vi "XGT 연속읽기 (독립).vi"() -> ()   [LabVIEW 2014]
uses:
  <vilib>/Instr/_visa.llb/VISA Configure Serial Port (Instr).vi
panel:
  out "error out":errorcluster
  in  "Start":bool
  out "배열":i32[](array[numeric])
  out "Array":i32[](array[numeric])
  in  "Address":string[](array[string])
  in  "length":i32=6
  out "데이터 개수":string
  out "에러 코드":string
  out "Waveform Graph":dbl[](graph)
  out "Serial Settings:Number of Bytes at Serial Port":u32
  in  "stop bits (10: 1 bit)":u16(ring)=10 caption="정지 비트(10: 1비트)" items=["1.0"=10, "1.5"=15, "2.0"=20]
  in  "parity (0:none)":enum16{"None", "Odd", "Even", "Mark", "Space"}(ring) caption="패리티(0:없음)"
  in  "data bits (8)":u16=8 caption="데이터 비트(8)" min=5 max=8 step=1
  in  "baud rate (9600)":u32=115200 caption="보 전송속도(9600)"
  in  "VISA resource name":refnum<visa-resource-name>="COM4" caption="VISA 리소스 이름"
  # "응답"
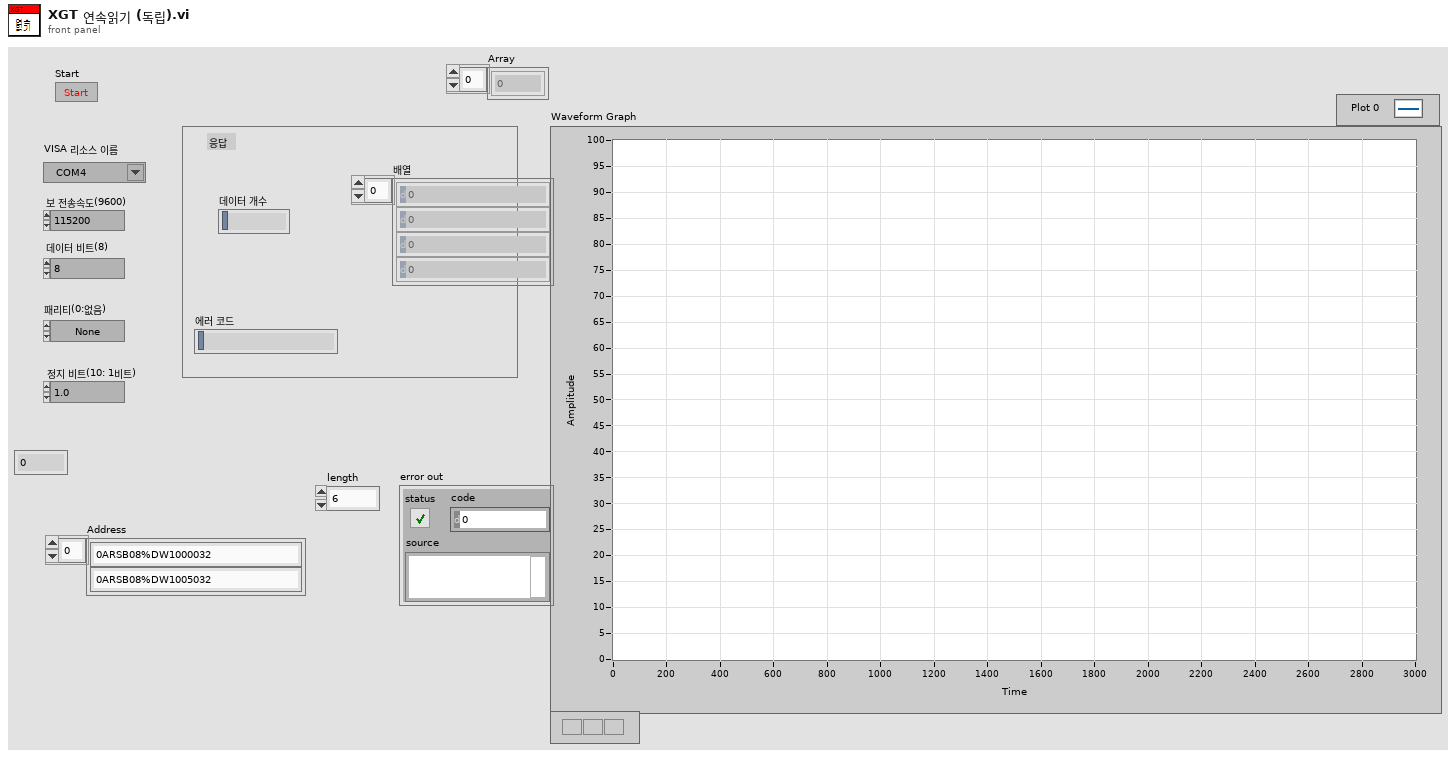
[diagram p1: front panel]
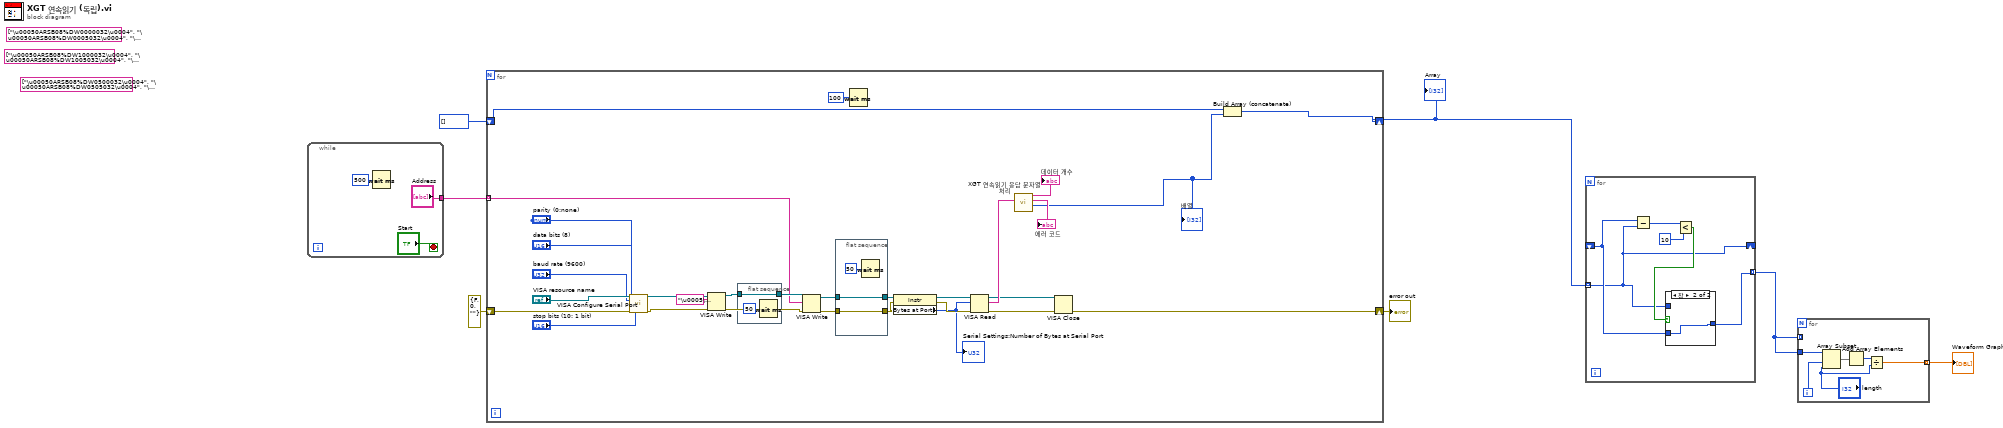
[diagram p0: block diagram]
diagram:
  (unwired) string[] ["\u00050ARSB08%DW1000032\u0004", "\u00050ARSB08%DW1005032\u0004", "\u00050ARSB08%DW1010032\u0004", "\u00050ARSB08%DW1015032\u0004", "\u00050ARSB08%DW1020032\u0004", "\u00050ARSB08%DW1025032\u0004", "\u00050ARSB08%DW1030032\u0004", "\u00050ARSB08%DW1035032\u0004", "\u00050ARSB08%DW1040032\u0004", "\u00050ARSB08%DW1045032\u0004", "\u00050ARSB08%DW1050032\u0004", "\u00050ARSB08%DW1055032\u0004", "\u00050ARSB08%DW1060032\u0004", "\u00050ARSB08%DW1065032\u0004", "\u00050ARSB08%DW1070032\u0004", "\u00050ARSB08%DW1075032\u0004", "\u00050ARSB08%DW1080032\u0004", "\u00050ARSB08%DW1085032\u0004", "\u00050ARSB08%DW1090032\u0004", "\u00050ARSB08%DW1095032\u0004", "\u00050ARSB08%DW1100032\u0004", "\u00050ARSB08%DW1105032\u0004", "\u00050ARSB08%DW1110032\u0004", "\u00050ARSB08%DW1115032\u0004", "\u00050ARSB08%DW1120032\u0004", "\u00050ARSB08%DW1125032\u0004", "\u00050ARSB08%DW1130032\u0004", "\u00050ARSB08%DW1135032\u0004", "\u00050ARSB08%DW1140032\u0004", "\u00050ARSB08%DW1145032\u0004", "\u00050ARSB08%DW1150032\u0004", "\u00050ARSB08%DW1155032\u0004", "\u00050ARSB08%DW1160032\u0004", "\u00050ARSB08%DW1165032\u0004", "\u00050ARSB08%DW1170032\u0004", "\u00050ARSB08%DW1175032\u0004", "\u00050ARSB08%DW1180032\u0004", "\u00050ARSB08%DW1185032\u0004", "\u00050ARSB08%DW1190032\u0004", "\u00050ARSB08%DW1195032\u0004", "\u00050ARSB08%DW1200032\u0004", "\u00050ARSB08%DW1205032\u0004", "\u00050ARSB08%DW1210032\u0004", "\u00050ARSB08%DW1215032\u0004", "\u00050ARSB08%DW1220032\u0004", "\u00050ARSB08%DW1225032\u0004", "\u00050ARSB08%DW1230032\u0004", "\u00050ARSB08%DW1235032\u0004", "\u00050ARSB08%DW1240032\u0004", "\u00050ARSB08%DW1245032\u0004", "\u00050ARSB08%DW1250032\u0004", "\u00050ARSB08%DW1255032\u0004", "\u00050ARSB08%DW1260032\u0004", "\u00050ARSB08%DW1265032\u0004", "\u00050ARSB08%DW1270032\u0004", "\u00050ARSB08%DW1275032\u0004", "\u00050ARSB08%DW1280032\u0004", "\u00050ARSB08%DW1285032\u0004", "\u00050ARSB08%DW1290032\u0004", "\u00050ARSB08%DW1295032\u0004"] ("Array")
  (unwired) string[] ["\u00050ARSB08%DW0500032\u0004", "\u00050ARSB08%DW0505032\u0004", "\u00050ARSB08%DW0510032\u0004", "\u00050ARSB08%DW0515032\u0004", "\u00050ARSB08%DW0520032\u0004", "\u00050ARSB08%DW0525032\u0004", "\u00050ARSB08%DW0530032\u0004", "\u00050ARSB08%DW0535032\u0004", "\u00050ARSB08%DW0540032\u0004", "\u00050ARSB08%DW0545032\u0004", "\u00050ARSB08%DW0550032\u0004", "\u00050ARSB08%DW0555032\u0004", "\u00050ARSB08%DW0560032\u0004", "\u00050ARSB08%DW0565032\u0004", "\u00050ARSB08%DW0570032\u0004", "\u00050ARSB08%DW0575032\u0004", "\u00050ARSB08%DW0580032\u0004", "\u00050ARSB08%DW0585032\u0004", "\u00050ARSB08%DW0590032\u0004", "\u00050ARSB08%DW0595032\u0004", "\u00050ARSB08%DW0600032\u0004", "\u00050ARSB08%DW0605032\u0004", "\u00050ARSB08%DW0610032\u0004", "\u00050ARSB08%DW0615032\u0004", "\u00050ARSB08%DW0620032\u0004", "\u00050ARSB08%DW0625032\u0004", "\u00050ARSB08%DW0630032\u0004", "\u00050ARSB08%DW0635032\u0004", "\u00050ARSB08%DW0640032\u0004", "\u00050ARSB08%DW0645032\u0004", "\u00050ARSB08%DW0650032\u0004", "\u00050ARSB08%DW0655032\u0004", "\u00050ARSB08%DW0660032\u0004", "\u00050ARSB08%DW0665032\u0004", "\u00050ARSB08%DW0670032\u0004", "\u00050ARSB08%DW0675032\u0004", "\u00050ARSB08%DW0680032\u0004", "\u00050ARSB08%DW0685032\u0004", "\u00050ARSB08%DW0690032\u0004", "\u00050ARSB08%DW0695032\u0004", "\u00050ARSB08%DW0700032\u0004", "\u00050ARSB08%DW0705032\u0004", "\u00050ARSB08%DW0710032\u0004", "\u00050ARSB08%DW0715032\u0004", "\u00050ARSB08%DW0720032\u0004", "\u00050ARSB08%DW0725032\u0004", "\u00050ARSB08%DW0730032\u0004", "\u00050ARSB08%DW0735032\u0004", "\u00050ARSB08%DW0740032\u0004", "\u00050ARSB08%DW0745032\u0004", "\u00050ARSB08%DW0750032\u0004", "\u00050ARSB08%DW0755032\u0004", "\u00050ARSB08%DW0760032\u0004", "\u00050ARSB08%DW0765032\u0004", "\u00050ARSB08%DW0770032\u0004", "\u00050ARSB08%DW0775032\u0004", "\u00050ARSB08%DW0780032\u0004", "\u00050ARSB08%DW0785032\u0004", "\u00050ARSB08%DW0790032\u0004", "\u00050ARSB08%DW0795032\u0004"] ("Array")
  (unwired) string[] ["\u00050ARSB08%DW0000032\u0004", "\u00050ARSB08%DW0005032\u0004", "\u00050ARSB08%DW0010032\u0004", "\u00050ARSB08%DW0015032\u0004", "\u00050ARSB08%DW0020032\u0004", "\u00050ARSB08%DW0025032\u0004", "\u00050ARSB08%DW0030032\u0004", "\u00050ARSB08%DW0035032\u0004", "\u00050ARSB08%DW0040032\u0004", "\u00050ARSB08%DW0045032\u0004", "\u00050ARSB08%DW0050032\u0004", "\u00050ARSB08%DW0055032\u0004", "\u00050ARSB08%DW0060032\u0004", "\u00050ARSB08%DW0065032\u0004", "\u00050ARSB08%DW0070032\u0004", "\u00050ARSB08%DW0075032\u0004", "\u00050ARSB08%DW0080032\u0004", "\u00050ARSB08%DW0085032\u0004", "\u00050ARSB08%DW0090032\u0004", "\u00050ARSB08%DW0095032\u0004", "\u00050ARSB08%DW0100032\u0004", "\u00050ARSB08%DW0105032\u0004", "\u00050ARSB08%DW0110032\u0004", "\u00050ARSB08%DW0115032\u0004", "\u00050ARSB08%DW0120032\u0004", "\u00050ARSB08%DW0125032\u0004", "\u00050ARSB08%DW0130032\u0004", "\u00050ARSB08%DW0135032\u0004", "\u00050ARSB08%DW0140032\u0004", "\u00050ARSB08%DW0145032\u0004", "\u00050ARSB08%DW0150032\u0004", "\u00050ARSB08%DW0155032\u0004", "\u00050ARSB08%DW0160032\u0004", "\u00050ARSB08%DW0165032\u0004", "\u00050ARSB08%DW0170032\u0004", "\u00050ARSB08%DW0175032\u0004", "\u00050ARSB08%DW0180032\u0004", "\u00050ARSB08%DW0185032\u0004", "\u00050ARSB08%DW0190032\u0004", "\u00050ARSB08%DW0195032\u0004", "\u00050ARSB08%DW0200032\u0004", "\u00050ARSB08%DW0205032\u0004", "\u00050ARSB08%DW0210032\u0004", "\u00050ARSB08%DW0215032\u0004", "\u00050ARSB08%DW0220032\u0004", "\u00050ARSB08%DW0225032\u0004", "\u00050ARSB08%DW0230032\u0004", "\u00050ARSB08%DW0235032\u0004", "\u00050ARSB08%DW0240032\u0004", "\u00050ARSB08%DW0245032\u0004", "\u00050ARSB08%DW0250032\u0004", "\u00050ARSB08%DW0255032\u0004", "\u00050ARSB08%DW0260032\u0004", "\u00050ARSB08%DW0265032\u0004", "\u00050ARSB08%DW0270032\u0004", "\u00050ARSB08%DW0275032\u0004", "\u00050ARSB08%DW0280032\u0004", "\u00050ARSB08%DW0285032\u0004", "\u00050ARSB08%DW0290032\u0004", "\u00050ARSB08%DW0295032\u0004"] ("Array")
  n1 = while {
    tunnel: ["Address"] -> w3
    stop <- "Start" stop-if-true
    n2 = Wait (ms)(milliseconds to wait=u32 500) -> ()  [unwired: 1 out]
  }
  n3 = for {
    tunnel: w3 -> [w16] mode=indexing
    shift-right: [w14] -> w5
    shift-left: i32[] [] -> [w13]
    shift-right: [w12] -> w1
    shift-left: errorcluster {"status"=FALSE, "code"=0, "source"=""} ("error out") -> [w11]
    n4 = call-poly "VISA Configure Serial Port"("VISA resource name"="VISA resource name", "baud rate (9600)"="baud rate (9600)", "data bits (8)"="data bits (8)", "parity (0:none)"="parity (0:none)", "error in (no error)"=w11, "stop bits (10: 1 bit)"="stop bits (10: 1 bit)") -> ("VISA resource name out"=w25:refnum<visa-resource-name>, "error out"=w24:errorcluster)  [unwired: 8 in]
    n5 = VISA Write(VISA resource name=w25, write buffer="\u0005\u0004", error in (no error)=w24) -> (VISA resource name out=w22:refnum<visa-resource-name>, error out=w23:errorcluster)  [unwired: 1 out]
    n6 = flat-sequence {
      tunnel: w22 -> [w42]
      tunnel: [w42] -> w21
      frame #0 {
        n7 = Wait (ms)(milliseconds to wait=u32 50) -> ()  [unwired: 1 out]
      }
    }
    n8 = VISA Write(VISA resource name=w21, write buffer=w16, error in (no error)=w23) -> (VISA resource name out=w39:refnum<visa-resource-name>, error out=w40:errorcluster)  [unwired: 1 out]
    n9 = flat-sequence {
      tunnel: w40 -> [w45]
      tunnel: [w45] -> w36
      tunnel: w39 -> [w44]
      tunnel: [w44] -> w37
      frame #0 {
        n10 = Wait (ms)(milliseconds to wait=u32 50 ("대기 시간(ms)")) -> ()  [unwired: 1 out]
      }
    }
    n11 = Wait (ms)(milliseconds to wait=u32 100 ("대기 시간(ms)")) -> ()  [unwired: 1 out]
    n12 = property class="Instr"(reference=w37, error in=w36) -> (reference out=w35:refnum<visa-resource-name>, error out=w38:errorcluster, "Bytes at Port"=w34:u32)
    "Serial Settings:Number of Bytes at Serial Port" <- w34
    n13 = VISA Read(VISA resource name=w35, byte count=w34, error in (no error)=w38) -> (VISA resource name out=w32:refnum<visa-resource-name>, read buffer=w33:string, error out=w26:errorcluster)  [unwired: 1 out]
    n14 = call "XGT 연속읽기 응답 문자열 처리.vi"("응답"=w33) -> ("배열"=w15:i32[], "에러 코드"=→"에러 코드":string, "데이터 개수"=→"데이터 개수":string)  [unwired: 5 in, 3 out]
    "배열" <- w15
    n15 = VISA Close(VISA resource name=w32, error in (no error)=w26) -> (error out=w12:errorcluster)
    n16 = Build Array (concatenate)(w13, w15) -> (w14:i32[])
  }
  "Array" <- w5
  "error out" <- w1
  n17 = for {
    tunnel: w5 -> [w47] mode=indexing
    tunnel: [w51] -> w6 mode=indexing
    shift-right: [w47] -> _
    shift-left: _ -> [w50]
    n18 = Subtract(x=w50, y=w47) -> (x-y=w46:i32)
    n19 = Less?(x=w46, y=10) -> (x < y?=w48:bool)
    n20 = case shown="참" w48 {
      tunnel: w47 -> [w52 _]
      tunnel: w50 -> [_ w53]
      tunnel: [w52 w53] -> w51
      frame False {
      }
      frame True {
      }
    }
  }
  n21 = for {
    tunnel: w6 -> [w59]
    tunnel: [w54] -> w4 mode=indexing
    tunnel: w6 -> [_] mode=indexing
    i -> [w58]
    n22 = Array Subset(array=w59, index=w58, length="length") -> (w57:i32[])
    n23 = Add Array Elements(numeric array=w57) -> (sum=w56:i32)
    n24 = Divide(x=w56, y="length") -> (x/y=w54:dbl)
  }
  "Waveform Graph" <- w4
